vi "PH_Beckhoff_StepMot.declare digital InputTags.vi"(3 "Instance Name":string="N/A") -> (0 "Digital Inputs":T1, 1 "Description":string)   [LabVIEW 2014, in "PH_Beckhoff_StepMot.lvlib"]
uses:
  PH_Beckhoff_StepMot.lvlib
  PH_Beckhoff/PH_Beckhoff.Digital Inputs.ctl
  PH_Beckhoff/PH_Beckhoff.lvlib
panel:
  out "Right Size?":bool
  # "Let this VI run to check the size!"
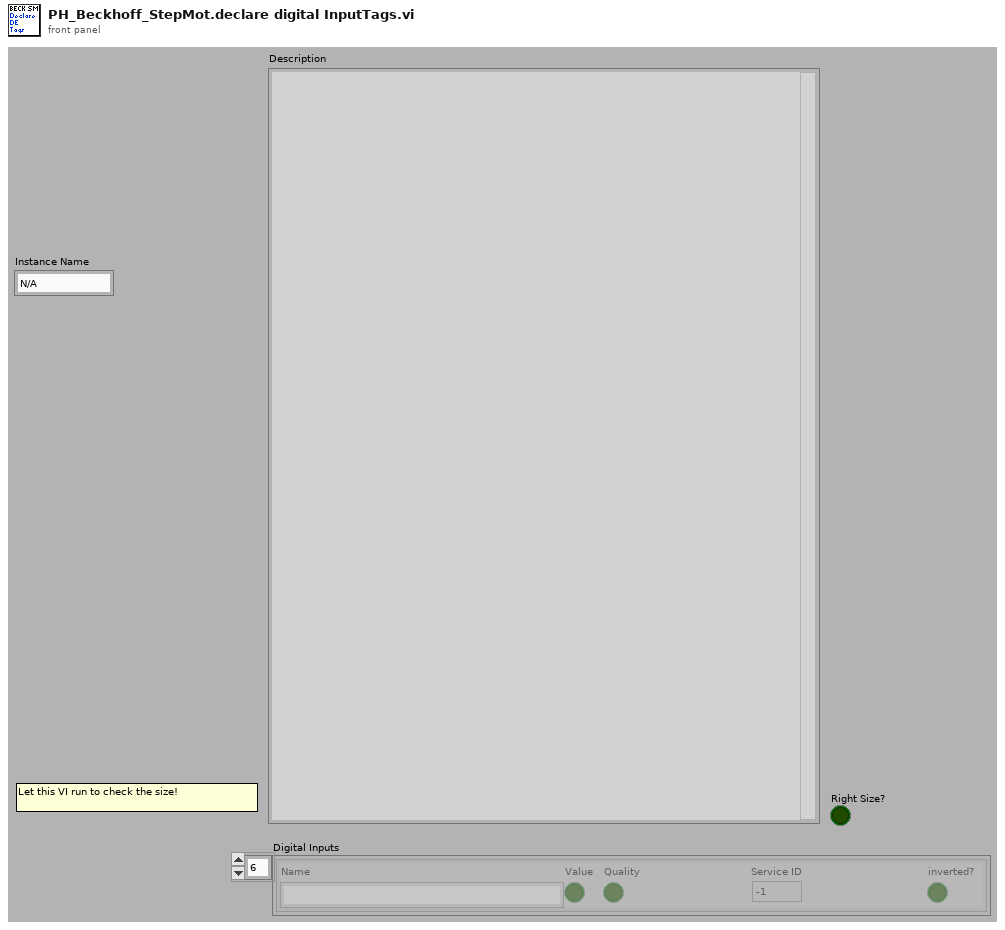
[diagram p1: front panel]
types:
  T1 = typedef "PH_Beckhoff.lvlib/PH_Beckhoff.Digital Inputs.ctl" = cluster{"Name":string, "Value":bool, "Quality":bool, "Service ID":i32, "inverted?":bool}[]
  T2 = cluster{"Name":string, "Value":bool, "Quality":bool, "Service ID":i32, "inverted?":bool}
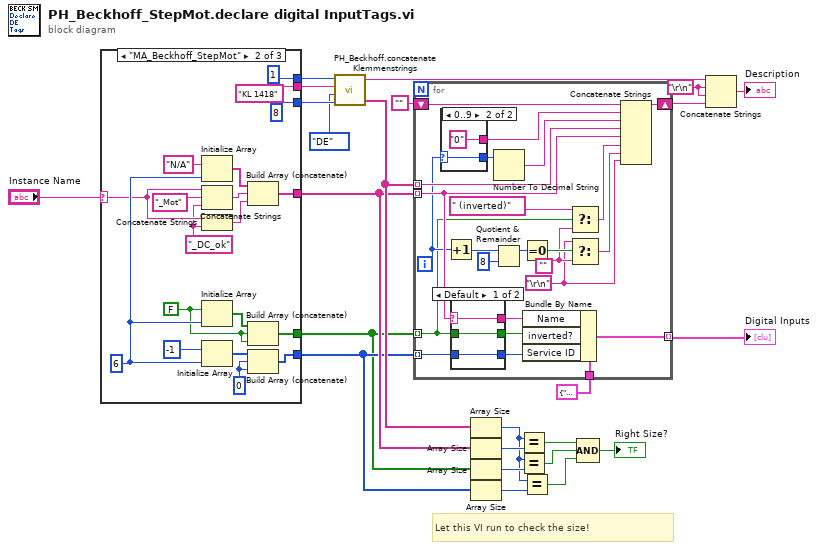
[diagram p0: block diagram]
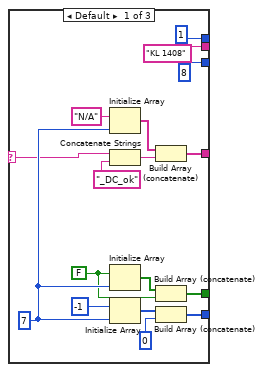
[diagram p2: hidden frame]
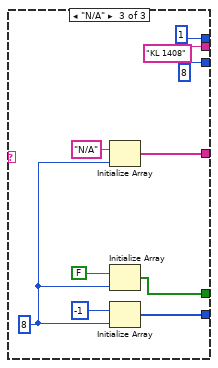
[diagram p3: hidden frame]
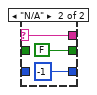
[diagram p4: hidden frame]
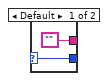
[diagram p5: hidden frame]
diagram:
  w22 = "\r\n"
  # "Let this VI run to check the size!"
  n1 = case shown="\"MA_Beckhoff_StepMot\"" "Instance Name" {
    selector: "Instance Name" -> [w25 w45 _]
    tunnel: ["KL 1408" ("Klemmenname") "KL 1418" ("Klemmenname") "KL 1408" ("Klemmenname")] -> w20
    tunnel: [8 ("# of In- or Outputs") 8 ("# of In- or Outputs") 8 ("# of In- or Outputs")] -> w19
    tunnel: [w35 w55 w61] -> w5
    tunnel: [w30 w51 w63] -> w4
    tunnel: [1 ("Quantity") 1 ("Quantity") 1 ("Quantity")] -> w3
    tunnel: [w27 w48 w62] -> w2
    frame Default {
      w33 = 7 ("dimension size")
      w26 = FALSE
      n2 = Initialize Array("N/A" ("string"), w33) -> (w36:string[])
      n3 = Concatenate Strings(w25, "_DC_ok" ("string")) -> (w38:string)
      n4 = Initialize Array(w26, w33) -> (w28:bool[])
      n5 = Initialize Array(-1 ("Service ID"), w33) -> (w32:i32[])
      n6 = Build Array (concatenate)(w36, w38) -> (w35:string[])
      n7 = Build Array (concatenate)(w28, w26) -> (w27:bool[])
      n8 = Build Array (concatenate)(w32, 0 ("Service ID")) -> (w30:i32[])
    }
    frame "MA_Beckhoff_StepMot" {
      w43 = 0 ("Service ID")
      w53 = 6 ("dimension size")
      w42 = FALSE
      w44 = "_DC_ok" ("string")
      n9 = Initialize Array("N/A" ("string"), w53) -> (w56:string[])
      n10 = Concatenate Strings(w45, "_Mot" ("string"), w44) -> (w47:string)
      n11 = Concatenate Strings(w45, w44) -> (w58:string)
      n12 = Initialize Array(w42, w53) -> (w49:bool[])
      n13 = Initialize Array(-1 ("Service ID"), w53) -> (w52:i32[])
      n14 = Build Array (concatenate)(w56, w47, w58) -> (w55:string[])
      n15 = Build Array (concatenate)(w49, w42, w42) -> (w48:bool[])
      n16 = Build Array (concatenate)(w52, w43, w43) -> (w51:i32[])
    }
    frame "N/A" {
      w66 = 8 ("dimension size")
      n17 = Initialize Array("N/A" ("string"), w66) -> (w61:string[])
      n18 = Initialize Array(FALSE, w66) -> (w62:bool[])
      n19 = Initialize Array(-1 ("Service ID"), w66) -> (w63:i32[])
    }
  }
  n20 = call "PH_Beckhoff.concatenate Klemmenstrings.vi"("# of In- or Outputs"=w19, "Type"=enum16{"AE", "AA", "DE", "DA", "SE"}."DE", "Klemmenname"=w20, "Quantity"=w3) -> ("concatenated string array"=w17:string[], "\"<Type>: <Quantity> x <Klemmenname>\""=w18:string)  [unwired: 1 out]
  n21 = for {
    tunnel: w5 -> [w87] mode=indexing
    tunnel: w17 -> [w91] mode=indexing
    shift-right: [w73] -> w23
    shift-left: "" -> [w74]
    tunnel: w2 -> [w78] mode=indexing
    tunnel: [w89] -> w10 mode=indexing
    tunnel: T2 {"Name"="", "Value"=FALSE, "Quality"=FALSE, "Service ID"=0, "inverted?"=FALSE} ("Digital Input Value") -> [w90]
    tunnel: w4 -> [w84] mode=indexing
    i -> [w83]
    w71 = "\r\n"
    w77 = ""
    n22 = case shown="0..9" w83 {
      selector: w83 -> [w101 w104]
      tunnel: [w101 w104] -> w94
      tunnel: ["" "0"] -> w93
      frame Default {
      }
      frame 0..9 {
      }
    }
    n23 = Increment(x=w83) -> (x+1=w82:i32)
    n24 = case shown="Default" w87 {
      selector: w87 -> [w95 w98]
      tunnel: w84 -> [w97 _]
      tunnel: [w97 -1 ("Service ID")] -> w86
      tunnel: w78 -> [w96 _]
      tunnel: [w96 FALSE ("element")] -> w85
      tunnel: [w95 w98] -> w88
      frame Default {
      }
      frame "N/A" {
      }
    }
    n25 = Number To Decimal String(number=w94) -> (decimal integer string=w92:string)  [unwired: 1 in]
    n26 = Quotient & Remainder(x=w82, y=8) -> (x-y*floor(x/y)=w80:i32)  [unwired: 1 out]
    n27 = Equal To 0?(x=w80) -> (x = 0?=w79:bool)
    n28 = Bundle By Name(cluster=w90, "Name"=w88, "inverted?"=w85, "Service ID"=w86) -> (w89:T2)
    n29 = Select(t=" (inverted)" ("string"), s=w78, f=w77) -> (s? t:f=w75:string)
    n30 = Select(t=w71, s=w79, f=w77) -> (s? t:f=w72:string)
    n31 = Concatenate Strings(w74, w93, w92, w91, w87, w75, w72, w71) -> (w73:string)
  }
  "Digital Inputs" <- w10
  n32 = Array Size(array=w17) -> (size(s)=w7:i32)
  n33 = Array Size(array=w5) -> (size(s)=w16:i32)
  n34 = Array Size(array=w2) -> (size(s)=w15:i32)
  n35 = Array Size(array=w4) -> (size(s)=w8:i32)
  n36 = Equal?(x=w7, y=w16) -> (x = y?=w13:bool)
  n37 = Equal?(x=w7, y=w15) -> (x = y?=w12:bool)
  n38 = Equal?(x=w7, y=w8) -> (x = y?=w6:bool)
  n39 = Compound Arithmetic op=AND(w13, w12, w6) -> (→"Right Size?":bool)
  n40 = Concatenate Strings(w18, w22, w22, w23) -> (→"Description":string)
